vi "PointByPointDifferentiation.vi"(8 "error in (no error)":errorcluster, 10 "Differentiation":T1={"Conversion Op"=enum."singleInt", "Unit"="", "Parent Unit"=""}, 11 "Waveform":waveform(sgl)) -> (0 "error out":errorcluster, 3 "Differentiated Waveform":waveform(sgl))   [LabVIEW 2017, in "CmsVirtualChannel.lvlib"]
uses:
  <vilib>/addons/InsightCM/Devices/Shared/Cms/CmsVirtualChannel/CmsVirtualChannel.lvlib
  <vilib>/addons/InsightCM/Devices/Shared/Cms/CmsVirtualChannel/controls/Differentiation.ctl
  <vilib>/addons/InsightCM/Utilities/Analysis/Shared/controls/ConversionOp.ctl
  <vilib>/addons/InsightCM/Utilities/Analysis/Vibration/VibrationAnalysisFunctions.lvlib
  <vilib>/addons/InsightCM/Utilities/Analysis/Shared/AnalysisHelper.lvlib
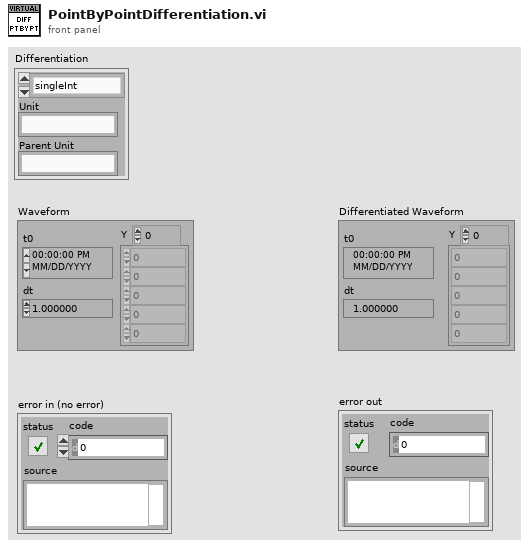
[diagram p1: front panel]
types:
  T1 = typedef "CmsVirtualChannel.lvlib/Differentiation.ctl" = cluster{"Conversion Op":T2, "Unit":string, "Parent Unit":string}
  T2 = typedef "AnalysisHelper.lvlib/ConversionOp.ctl" = enum16{"none", "singleInt", "doubleInt", "singleDiff", "doubleDiff"}
  T3 = enum16{"single integration", "double integration", "single differentiation", "double differentiation", "none"}
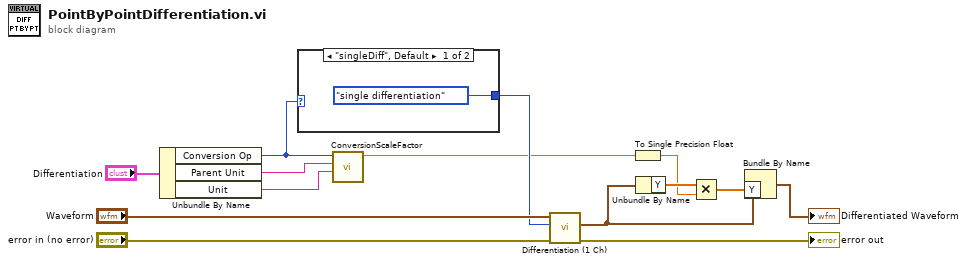
[diagram p0: block diagram]
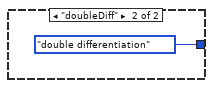
[diagram p2: hidden frame]
diagram:
  n1 = Unbundle By Name("Differentiation") -> ("Conversion Op"=w5:T2, "Parent Unit"=w4:string, "Unit"=w3:string)
  n2 = case shown="\"singleDiff\", Default" w5 {
    tunnel: [T3."single differentiation" ("integration type") T3."double differentiation" ("integration type")] -> w11
    frame "singleDiff", Default {
    }
    frame "doubleDiff" {
    }
  }
  n3 = call <vilib>:"ConversionScaleFactor.vi"("Desired Unit"=w3, "Original Unit"=w4, "Conversion Op"=w5) -> ("Scale Factor"=w2:dbl)  [unwired: 8 in]
  n4 = call <vilib>:"Differentiation (1 Ch).vi"("error in (no error)"="error in (no error)", "differentiation type"=w11, "Signal"="Waveform") -> ("error out"=→"error out":errorcluster, "Differentiated Signal"=w10:waveform(sgl))  [unwired: 7 in]
  n5 = To Single Precision Float(number=w2) -> (single precision float=w1:sgl)
  n6 = Unbundle By Name(w10) -> ("Y"=w9:sgl[])
  n7 = Multiply(x=w9, y=w1) -> (x*y=w8:sgl[])
  n8 = Bundle By Name(cluster=w10, "Y"=w8) -> (→"Differentiated Waveform":waveform(sgl))
